vi "niFpgaDcRmsDefaultTemplate.vi"(0 "input data":fxp<+/-,16,16>, 1 "reset":bool) -> (4 "DC result":fxp<+/-,16,16>, 10 "results valid":bool)   [LabVIEW 2017]
uses:
  <vilib>/Platform/TimedLoop/XDataNode/timing_clust.ctl
  <vilib>/Platform/TimedLoop/XDataNode/nitl_modes.ctl
  <vilib>/Platform/TimedLoop/XDataNode/wakeup.ctl
  <vilib>/rvi/FXPMathLib/basic elements/FxpIntAccumulator/subVIs/nifxpmath_IntAccumulator_SimConfig.ctl
  <vilib>/rvi/FXPMathLib/basic elements/FxpIntAccumulator/simVIs/DllFxpIntAccumulator_sub.vi
  <vilib>/Platform/TimedLoop/XDataNode/XDataNode.xnode
  <vilib>/rvi/FXPMathLib/basic elements/FxpIntAccumulator/XNode/nifxpmath_IntAccumulator.xnode
  <vilib>/rvi/FXPMathLib/FxpMul/XNode/nifxpmath_Multiplier.xnode
  <vilib>/Platform/TimedLoop/XDataNode/XDNodeRunTimeDep.lvlib
  <vilib>/rvi/FXPMathLib/sim/FxpSim.dll
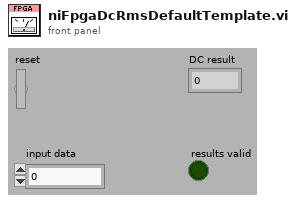
[diagram p1: front panel]
types:
  T1 = typedef "XDNodeRunTimeDep.lvlib/timing_clust.ctl" = cluster{"Expected End [f-1]":u64, "Actual End [f-1]":u64, "Finished Late? [f-1]":bool, "Expected End [i-1]":u64, "Actual End [i-1]":u64, "Finished Late? [i-1]":bool, "Expected Start [i]":u64, "Actual Start [i]":u64, "Expected Start [f]":u64, "Actual Start [f]":u64, "Source Name":string, "Structure Name":string, "Period":i64, "Deadline":i64, "Offset":i64, "Start":i64, "Priority":i32, "Timeout":i32, "Mode":T2, "Wakeup Reason":T3, "Error":errorcluster, "Source Type":string, "Secondary Source Type":string, "Global End Time":u64, "Global Start Time":u64, "Frame Duration":u64, "Iteration Duration":u64, "Assigned CPU":i32, "I/O Scan Engine Mode":u32}
  T2 = typedef "XDNodeRunTimeDep.lvlib/nitl_modes.ctl" = enum32{"No Change", "Process missed periods, maintain original phase", "Discard missed periods, maintain original phase", "Process missed periods, ignore original phase", "Discard missed periods, ignore original phase"}
  T3 = typedef "XDNodeRunTimeDep.lvlib/wakeup.ctl" = enum32{"Normal", "Aborted", "Asynchronous wakeup", "Timing source error", "Timed loop error", "Timeout"}
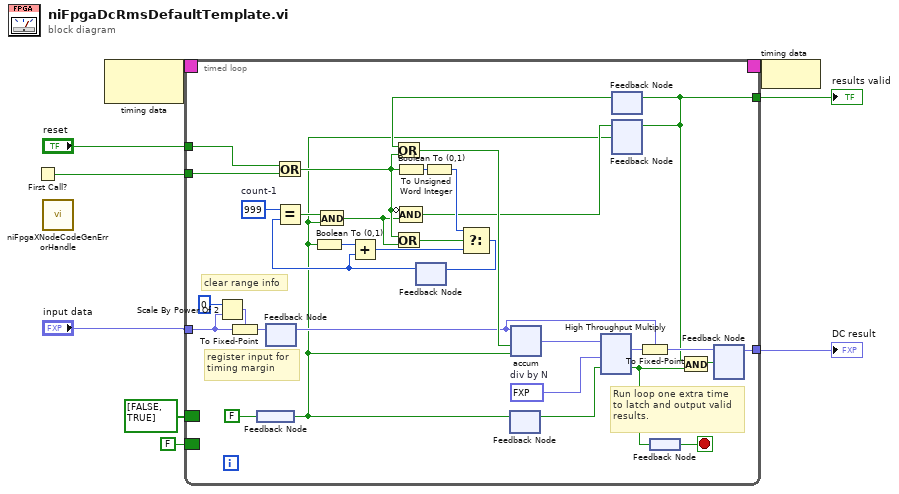
[diagram p0: block diagram]
diagram:
  n1 = First Call?() -> (First Call?: T/F=w7:bool)
  n2 = call <vilib>:"niFpgaXNodeCodeGenErrorHandle.vi"() -> ()  [unwired: 1 in]
  n3 = node-c288() -> (w6:T1)  [unwired: 1 in]
  n4 = timed-loop {
    tunnel: [w16] -> w9
    tunnel: "input data" -> [w11]
    tunnel: "reset" -> [w38]
    tunnel: w7 -> [w37]
    tunnel: [w15] -> w8
    timing: w6 -> [_]
    timing-out: [_] -> w5
    border: bool[] [FALSE, TRUE] -> [_]
    border: FALSE ("output valid") -> [_]
    stop <- w14 stop-if-true
    w28 = fxp<+,17,-9> 0.0010000020265579224  # div by N
    w42 = u16 999  # count-1
    # "Run loop one extra time\nto latch and output valid\nresults."
    # "register input for \ntiming margin"
    # "clear range info"
    n5 = Scale By Power Of 2(n=0, x=w11) -> (x*2^n=w21:fxp<+/-,16,16>)
    n6 = To Fixed-Point(fixed-point type=w21, number=w11) -> (fixed-point=w10:fxp<+/-,16,16>)
    n7 = feedback #1() -> (w18:bool)
    n8 = feedback-in #1(FALSE) -> ()
    n9 = feedback-in #2(w10) -> ()
    n10 = feedback #2() -> (w20:fxp<+/-,16,16>)  [unwired: 1 in]
    n11 = Or(x=w38, y=w37) -> (x .or. y?=w32:bool)
    n12 = Boolean To (0,1)(Boolean=w18) -> (0, 1=w36:i16)
    n13 = Boolean To (0,1)(Boolean=w32) -> (0, 1=w41:i16)
    n14 = feedback #3() -> (w29:u16)  [unwired: 1 in]
    n15 = Equal?(x=w42, y=w29) -> (x = y?=w34:bool)
    n16 = And(x=w34, y=w18) -> (x .and. y?=w31:bool)
    n17 = Add(x=w36, y=w29) -> (x+y=w35:u16)
    n18 = Or(x=w32, y=w31) -> (x .or. y?=w33:bool)
    n19 = Compound Arithmetic op=AND(invert w32, w31) -> (w24:bool)
    n20 = To Unsigned Word Integer(number=w41) -> (unsigned 16bit integer=w40:u16)
    n21 = Select(t=w40, s=w33, f=w35) -> (s? t:f=w39:u16)
    n22 = feedback-in #3(w39) -> ()
    n23 = feedback-in #4(w18) -> ()
    n24 = feedback #4() -> (w25:bool)  [unwired: 1 in]
    n25 = feedback #5() -> (w30:bool)  [unwired: 1 in]
    n26 = Or(x=w30, y=w32) -> (x .or. y?=w26:bool)
    n27 = xnode "accum"("x"=w20, "load (F)"=w26, "enable (T)"=w18) -> ("s"=w27:fxp<+/-,26,26>)  [unwired: 2 in, 1 out]
    n28 = xnode ("High Throughput Multiply")("x"=w27, "y"=w28, "input valid"=w25) -> ("x*y"=w23:fxp<+/-,43,17>, "output valid"=w12:bool)  [unwired: 1 in, 1 out]
    n29 = feedback-in #6(w24, w18) -> ()
    n30 = feedback #6() -> (w15:bool)  [unwired: 1 in]
    n31 = feedback-in #5(w15) -> ()
    n32 = To Fixed-Point(fixed-point type=w20, number=w23) -> (fixed-point=w17:fxp<+/-,16,16>)
    n33 = feedback #7() -> (w14:bool)
    n34 = feedback-in #7(w12) -> ()
    n35 = And(x=w15, y=w12) -> (x .and. y?=w13:bool)
    n36 = feedback #8() -> (w16:fxp<+/-,16,16>)  [unwired: 1 in]
    n37 = feedback-in #8(w17, w13) -> ()
  }
  "DC result" <- w9
  "results valid" <- w8
  n38 = node-c288(w5) -> ()
